vi "Settings Dialog.vi"(8 "error in (no error)":errorcluster, 11 "Settings in":T1) -> (0 "error out":errorcluster, 1 "Cancelled?":bool, 2 "UI Refresh Needed?":bool, 3 "Settings out":T1)   [LabVIEW 2025, in "Settings.lvlib"]
doc: "Dialog for selecting user specified settings."
uses:
  Settings.lvlib
  Settings.ctl
  Acquisition/Hardware Configuration.ctl
  Acquisition/Signal Type.ctl
  Logging/Logging Configuration.ctl
  <vilib>/Utility/xml.llb/Write to XML File(string).vi
  Acquisition/Acquisition.lvlib
  Logging/Logging.lvlib
panel:
  in  "Log File Path":path
  in  "Signal Type":u16(ring) items=["Sine Wave", "Square with Noise"]
  in  "Cancel Button":bool
  in  "OK Button":bool
  # "Non visible portion of dialog (needed for connector pane)."
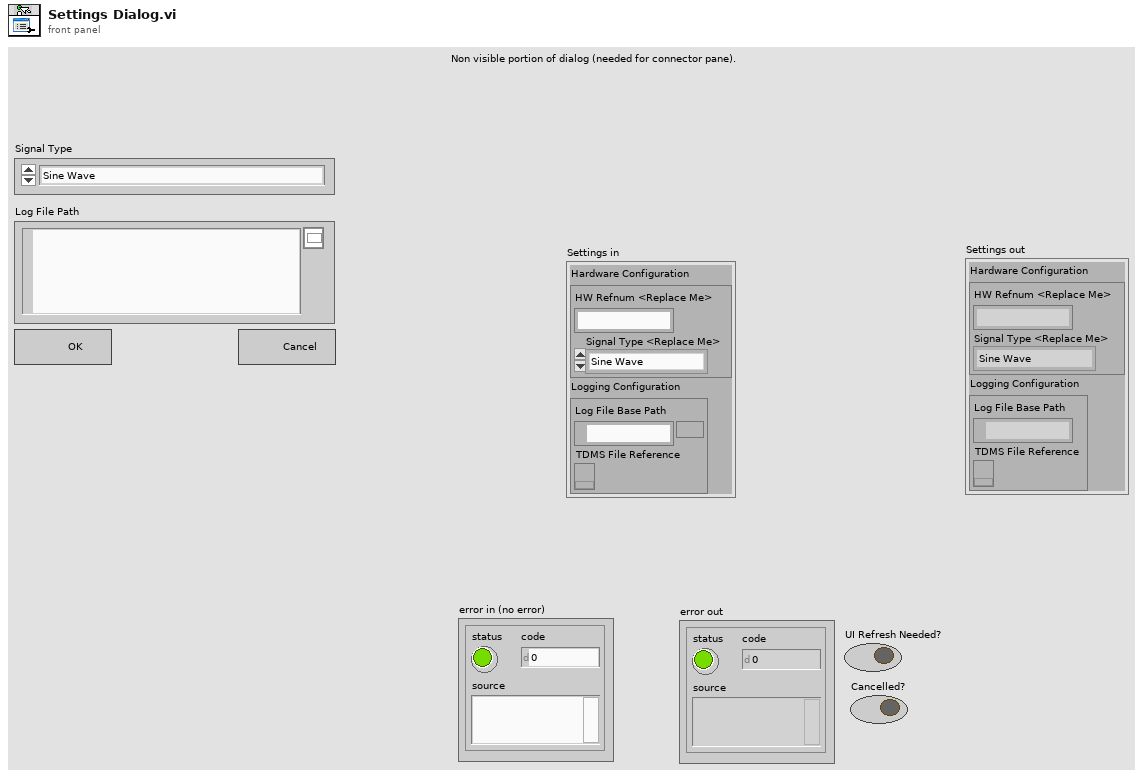
[diagram p1: front panel]
types:
  T1 = typedef "Settings.lvlib/Settings.ctl" = cluster{"Hardware Configuration":T2, "Logging Configuration":T4}
  T2 = typedef "Acquisition.lvlib/Hardware Configuration.ctl" = cluster{"HW Refnum <Replace Me>":string, "Signal Type <Replace Me>":T3}
  T3 = typedef "Acquisition.lvlib/Signal Type.ctl" = enum16{"Sine Wave", "Square with Noise"}
  T4 = typedef "Logging.lvlib/Logging Configuration.ctl" = cluster{"Log File Base Path":path, "TDMS File Reference":refnum<k34>}
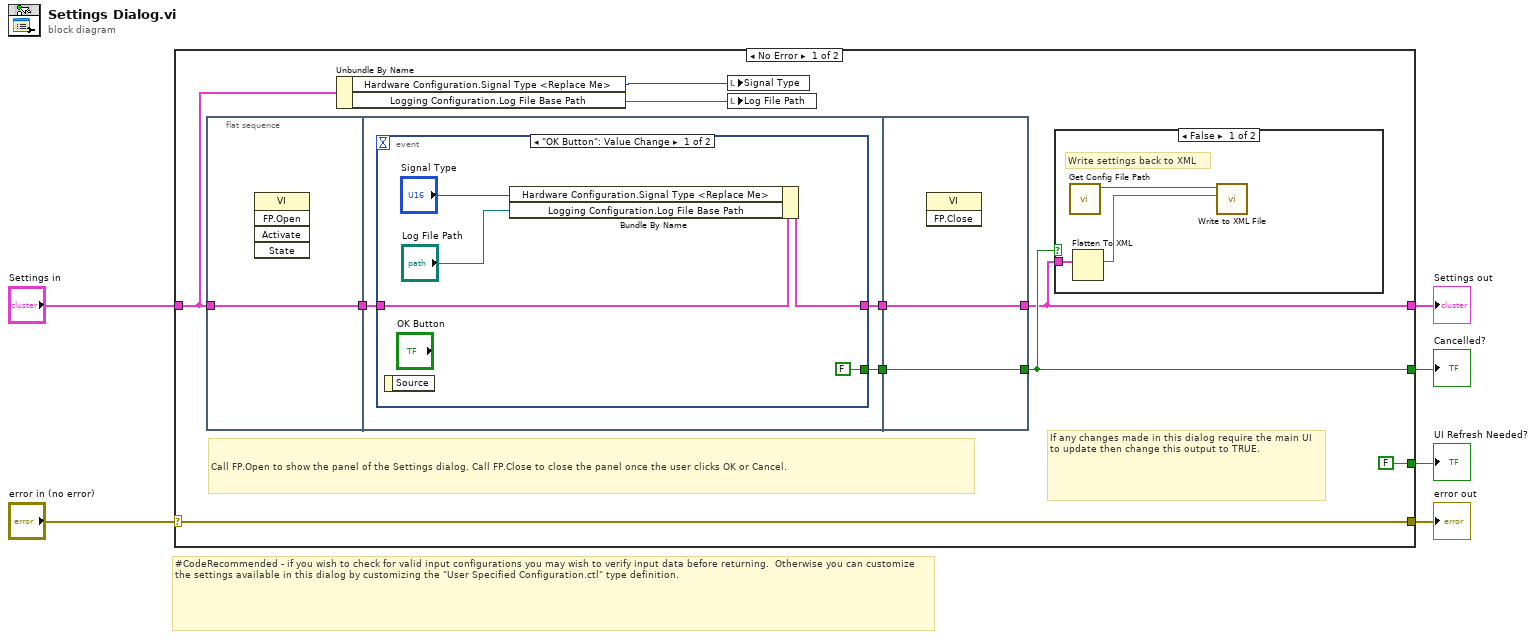
[diagram p0: block diagram]
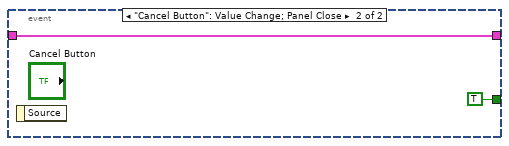
[diagram p2: hidden frame]
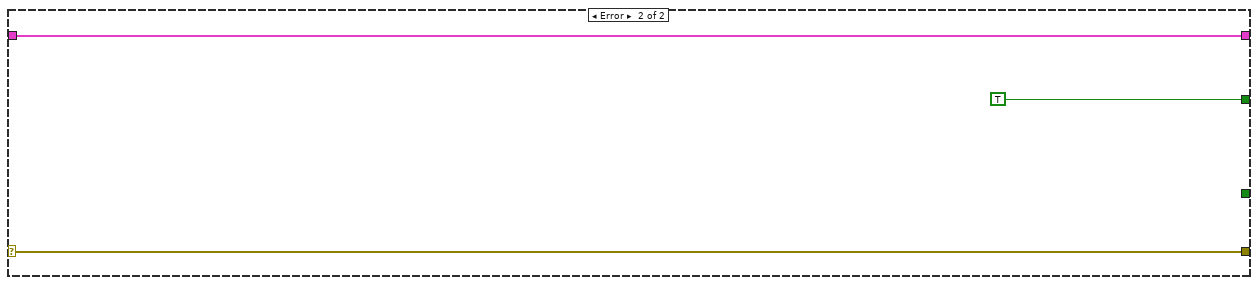
[diagram p4: hidden frame]
diagram:
  # "#CodeRecommended - if you wish to check for valid input configurations you may wish to verify input data before returning.  Otherwise you can customize the settings available in this dialog by customizing the \"User Specified Configuration.ctl\" type definition."
  n1 = case shown="No Error" "error in (no error)" {
    selector: "error in (no error)" -> [w16 w35]
    tunnel: [w16 w35] -> w5
    tunnel: "Settings in" -> [w12 w34]
    tunnel: [w13 w34] -> w3
    tunnel: [FALSE ("UI Refresh Needed?") _] -> w2
    tunnel: [w14 TRUE ("UI Refresh Needed?")] -> w1
    frame No Error {
      # "Call FP.Open to show the panel of the Settings dialog. Call FP.Close to close the panel once the user clicks OK or Cancel."
      # "If any changes made in this dialog require the main UI to update then change this output to TRUE."
      n2 = flat-sequence {
        tunnel: w12 -> [w17]
        tunnel: [w17] -> w9
        tunnel: w9 -> [w18]
        tunnel: [w20] -> w8
        tunnel: [w19] -> w7
        tunnel: [w28] -> w13
        tunnel: [w29] -> w14
        tunnel: w8 -> [w29]
        tunnel: w7 -> [w28]
        frame #0 {
          n3 = invoke class="VI" method="FP.Open"() -> ()  [unwired: 5 in, 5 out]
        }
        frame #1 {
          n4 = event shown="[0] \"OK Button\": Value Change" {
            selector: _ -> [_ _]
            dyn-events: _ -> [_ _]
            timeout: _ -> [_ _]
            tunnel: [w23 w27] -> w19
            tunnel: w18 -> [w24 w27]
            tunnel: [FALSE ("UI Refresh Needed?") TRUE ("UI Refresh Needed?")] -> w20
            event "OK Button": Value Change {
              n5 = event-data() -> ()  [unwired: 1 in, 1 out]
              n6 = Bundle By Name(cluster=w24, "Hardware Configuration.Signal Type <Replace Me>"="Signal Type", "Logging Configuration.Log File Base Path"="Log File Path") -> (w23:T1)
            }
            event "Cancel Button": Value Change; Panel Close {
              n7 = event-data() -> ()  [unwired: 1 in, 1 out]
            }
          }
        }
        frame #2 {
          n8 = invoke class="VI" method="FP.Close"() -> ()  [unwired: 3 in, 3 out]
        }
      }
      n9 = Unbundle By Name(w12) -> ("Hardware Configuration.Signal Type <Replace Me>"=w11:T3, "Logging Configuration.Log File Base Path"=w10:path)
      n10 = local write "Signal Type"(w11) -> ()
      n11 = local write "Log File Path"(w10) -> ()
      n12 = case shown="False" w14 {
        tunnel: w13 -> [w31 _]
        frame False {
          # "Write settings back to XML"
          n13 = call "Get Config File Path.vi"() -> ("XML File Path"=w32:path)  [unwired: 10 in, 1 out]
          n14 = Flatten To XML(6:w31) -> (2:w30:string)
          n15 = call-poly <vilib>:"Write to XML File.vi"("XML Input"=w30, "XML File Path"=w32) -> ()  [unwired: 7 in, 3 out]
        }
        frame True {
        }
      }
    }
    frame Error {
    }
  }
  "UI Refresh Needed?" <- w2
  "error out" <- w5
  "Settings out" <- w3
  "Cancelled?" <- w1
